vi "Read Frequency.vi"(11 "Signal Generator in":refnum<class "Signal Generator.lvclass">) -> (2 "Frequency":dbl, 3 "Signal Generator out":refnum<class "Signal Generator.lvclass">)   [LabVIEW 2020, in "Signal Generator.lvclass"]
uses:
  Signal Generator.lvclass
  Signal Generator.lvclass/Signal Generator.ctl
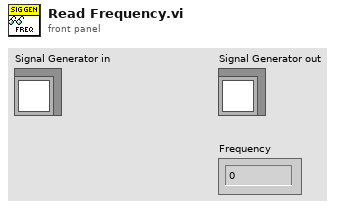
[diagram p1: front panel]
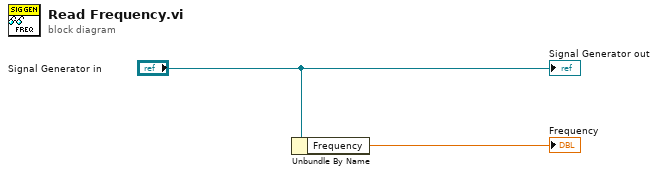
[diagram p0: block diagram]
diagram:
  n1 = Unbundle By Name("Signal Generator in") -> ("Frequency"=→"Frequency":dbl)
  "Signal Generator out" <- "Signal Generator in"
